vi "remove_lower_case.vi"(8 "error in (no error)":errorcluster, 11 "Instrument Command In":string=":TRIGger:PFERror[:SEQuence]:SOURce EXTernal[1]|EXTernal2|IMMediate|LINE|FRAMe|RFBurst|VIDeo,<freq>,<time>") -> (0 "error out":errorcluster, 3 "Instrument Command Out":string=":TRIG:PFER[:SEQ]:SOUR EXT[1]|EXT2|IMM|LINE|FRAM|RFB|VID,<FREQ>,<TIME>")   [LabVIEW 2018]
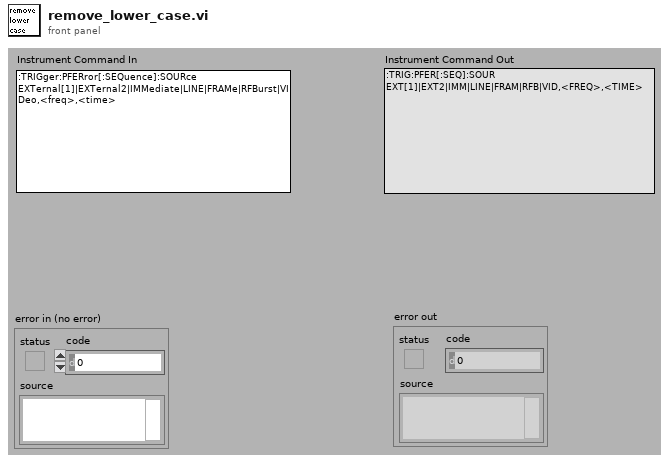
[diagram p1: front panel]
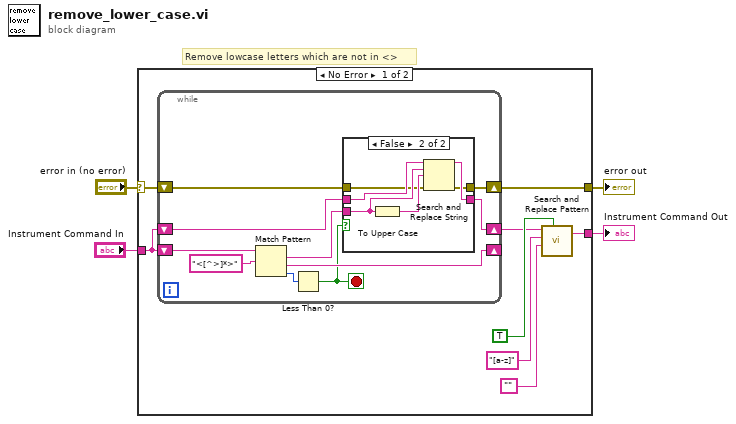
[diagram p0: block diagram]
diagram:
  # "Remove lowcase letters which are not in <>"
  n1 = case shown="No Error" "error in (no error)" {
    selector: "error in (no error)" -> [w6 w31]
    tunnel: [w9 w32] -> w4
    tunnel: "Instrument Command In" -> [w7 w32]
    tunnel: [w5 w31] -> w1
    frame No Error {
      n2 = while {
        shift-right: [w16] -> _
        shift-left: w7 -> [w21]
        shift-right: [w19] -> w8
        shift-left: w7 -> [w17]
        shift-right: [w13] -> w5
        shift-left: w6 -> [w14]
        stop <- w15 stop-if-true
        n3 = Match Pattern(string=w21, regular expression="<[^>]*>") -> (match substring=w20:string, after substring=w16:string, offset past match=w18:i32)  [unwired: 2 out]
        n4 = Less Than 0?(x=w18) -> (x < 0?=w15:bool)
        n5 = case shown="False" w15 {
          tunnel: w17 -> [w24 w30]
          tunnel: w20 -> [_ w29]
          tunnel: [w24 w27] -> w19
          tunnel: w14 -> [w23 w26]
          tunnel: [w23 w25] -> w13
          frame True {
          }
          frame False {
            n6 = To Upper Case(1:w29) -> (0:w28:string)
            n7 = Search and Replace String(input string=w30, search string=w29, replace string=w28, error in=w26) -> (result string=w27:string, error out=w25:errorcluster)  [unwired: 6 out]
          }
        }
      }
      n8 = call <vilib>:"Search and Replace Pattern.vi"("string"=w8, "regular expression (\"\")"="[a-z]" ("regular expression (\"\")"), "replace string (\"\")"="", "replace all? (F)"=TRUE) -> ("result string"=w9:string)  [unwired: 2 out]
    }
    frame Error {
    }
  }
  "Instrument Command Out" <- w4
  "error out" <- w1
